vi "Check for Errors.vi"(8 "error in (no error)":errorcluster, 10 "Preceding Items":refnum<class "Item.lvclass">[](array[class]), 11 "ZIP Item in":refnum<class "ZIP Item.lvclass">) -> (0 "error out":errorcluster, 2 "Error User Text":string)   [LabVIEW 2019, in "ZIP.lvlib" / "ZIP Item.lvclass"]
doc: "Checks the item for errors. This method is called a lot by the UI, so it should execute quickly.\n\nCopyright: MGI 2016\nAuthor: Derek Trepanier"
uses:
  ZIP Item.lvclass
  libs/Solution.lvlibp/Solution/Item/Item.lvclass
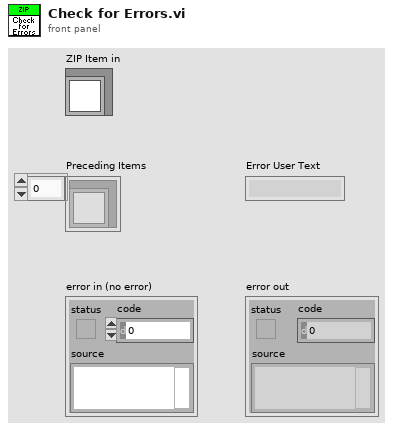
[diagram p1: front panel]
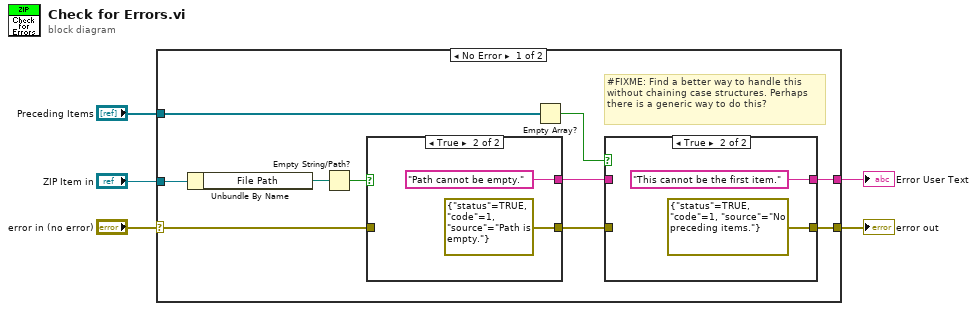
[diagram p0: block diagram]
diagram:
  n1 = case shown="No Error" "error in (no error)" {
    selector: "error in (no error)" -> [w12 w23]
    tunnel: "ZIP Item in" -> [w15 _]
    tunnel: [w6 w23] -> w4
    tunnel: [w7 _] -> w3
    tunnel: "Preceding Items" -> [w11 _]
    frame No Error {
      # "#FIXME: Find a better way to handle this without chaining case structures. Perhaps there is a generic way to do this?"
      n2 = Unbundle By Name(w15) -> ("File Path"=w14:path)
      n3 = Empty String/Path?(string/path=w14) -> (empty?=w13:bool)
      n4 = case shown="True" w13 {
        tunnel: [w20 errorcluster {"status"=TRUE, "code"=1, "source"="Path is empty."} ("error constant")] -> w10
        tunnel: [_ "Path cannot be empty." ("Error User Text")] -> w8
        tunnel: w12 -> [w20 _]
        frame False {
        }
        frame True {
        }
      }
      n5 = Empty Array?(array=w11) -> (empty?=w9:bool)
      n6 = case shown="True" w9 {
        tunnel: [w17 errorcluster {"status"=TRUE, "code"=1, "source"="No preceding items."} ("error constant")] -> w6
        tunnel: [w16 "This cannot be the first item." ("Error User Text")] -> w7
        tunnel: w10 -> [w17 _]
        tunnel: w8 -> [w16 _]
        frame False {
        }
        frame True {
        }
      }
    }
    frame Error {
    }
  }
  "error out" <- w4
  "Error User Text" <- w3
